vi "bson_iterator_init.vi"(10 "bson ptr":u32, 11 "bson_iterator ptr":u32) -> (2 "bson ptr out":u32, 3 "bson_iterator ptr out":u32)   [LabVIEW 2013]
uses:
  mongo-c-driver/libmongoc.so
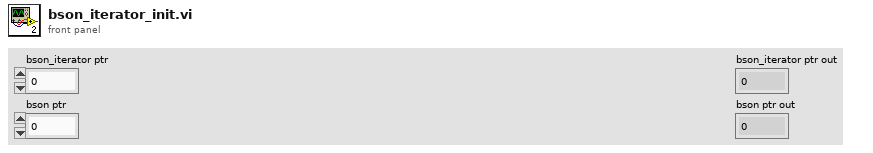
[diagram p1: front panel]
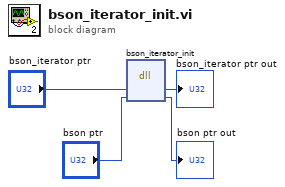
[diagram p0: block diagram]
diagram:
  n1 = dll-call lib="home/scot/dev/git/mongo-c-driver/libmongoc.so" fn="bson_iterator_init"("bson_iterator ptr"="bson_iterator ptr", "bson ptr"="bson ptr") -> ("bson_iterator ptr"=→"bson_iterator ptr out":u32, "bson ptr"=→"bson ptr out":u32)  [unwired: 4 in, 2 out]
